vi "testVI.vi"() -> ()   [LabVIEW 2012]
uses:
  <vilib>/measure/NI_MABase.lvlib
  pgfPlotAxis_tdef.ctl
  pgfPlotPlot_tdef.ctl
  <vilib>/Waveform/WDTOps.llb/WDT Get Waveform Time Array DBL.vi
panel:
  in  "png?":bool=TRUE
  out "standard output":string
  out "output png":picture
  in  "amplitude":dbl=21.0 format="%0.2p"
  in  "frequency":dbl=3.0 format="%0.2p"
  in  "signal type":T1(ring)=enum."Triangle Wave"
  in  "add noise":bool=TRUE
  in  "number of points":dbl(slide)=44.4776119402985 scale=10.0..1000.0
  out "LaTeX output":string
  out "Waveform Graph":waveform(dbl)[](graph)=[{"t0"=timestamp(0 s since 1904-01-01), "dt"=0.02248322147651007, "Y"=[-1.546477433388504, 4.661984807620563, 7.8278201832138725, 11.001512342104604, 15.015062026967165, 15.512826662722626, 15.574358460996109, 13.290410667596724, 11.99348612908547, 8.588629763986237, 5.067512693167407, 1.258457503857374, -2.8810456117563374, -6.925805192568073, -10.545354256767709, -14.932883970541788, -13.577918727803066, -14.589587562163713, -11.46193309140618, -12.290200153543955, -9.437814005181771, -4.8264367558785795, -1.2386574847111085, 3.051340081786596, 6.950914289149695, 9.981049349063406, 12.35566247672647, 15.294188005780697, 14.350046666102049, 14.978056870639572, 13.443684958705374, 9.524808574601101, 5.281310569613, 0.09035510962493731, -3.3367521947681373, -5.625031359450402, -10.134935689127893, -12.522309407667565, -13.59685597158344, -14.168685301718552, -14.20184362459651, -12.77561767255461, -10.526530375259396, -7.10442228803309]}, {"t0"=timestamp(0 s since 1904-01-01), "dt"=0.001, "Y"=array[1000 elements]}]
  in  "Amplitude":dbl(slide)=15.016835016835017 scale=0.0..20.0
  # "first signal"
  # "second signal"
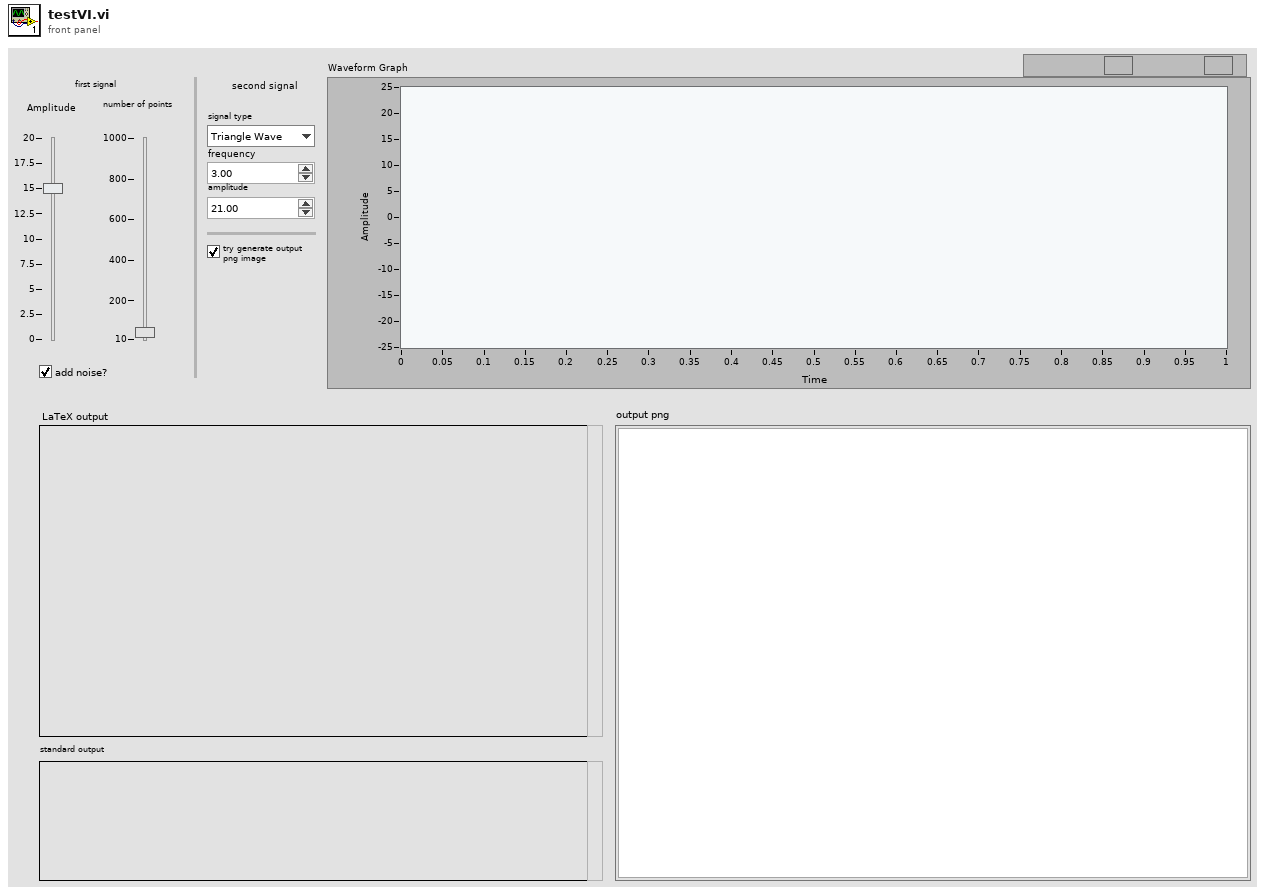
[diagram p1: front panel]
types:
  T1 = enum16{"Sine Wave", "Triangle Wave", "Square Wave", "Sawtooth Wave"}
  T2 = typedef "pgfPlotAxis_tdef.ctl" = cluster{"xmin":dbl, "xmax":dbl, "ymin":dbl, "ymax":dbl, "xLabel":string, "yLabel":string}
  T3 = typedef "pgfPlotPlot_tdef.ctl" = cluster{"LineStyle":u8, "LineWidth":u8, "PlotColor":u32, "Marker":u8, "PlotName":string, "x values":dbl[], "y values":dbl[]}
  T4 = typedef "LVBoundsTypeDef.ctl" = cluster{"Width":u32, "Height":u32}
  T5 = typedef "imagedata.ctl" = cluster{"image type":i32, "image depth":i32, "image":u8[], "mask":u8[], "colors":u32[], "Rectangle":cluster{"left":i16, "top":i16, "right":i16, "bottom":i16}}
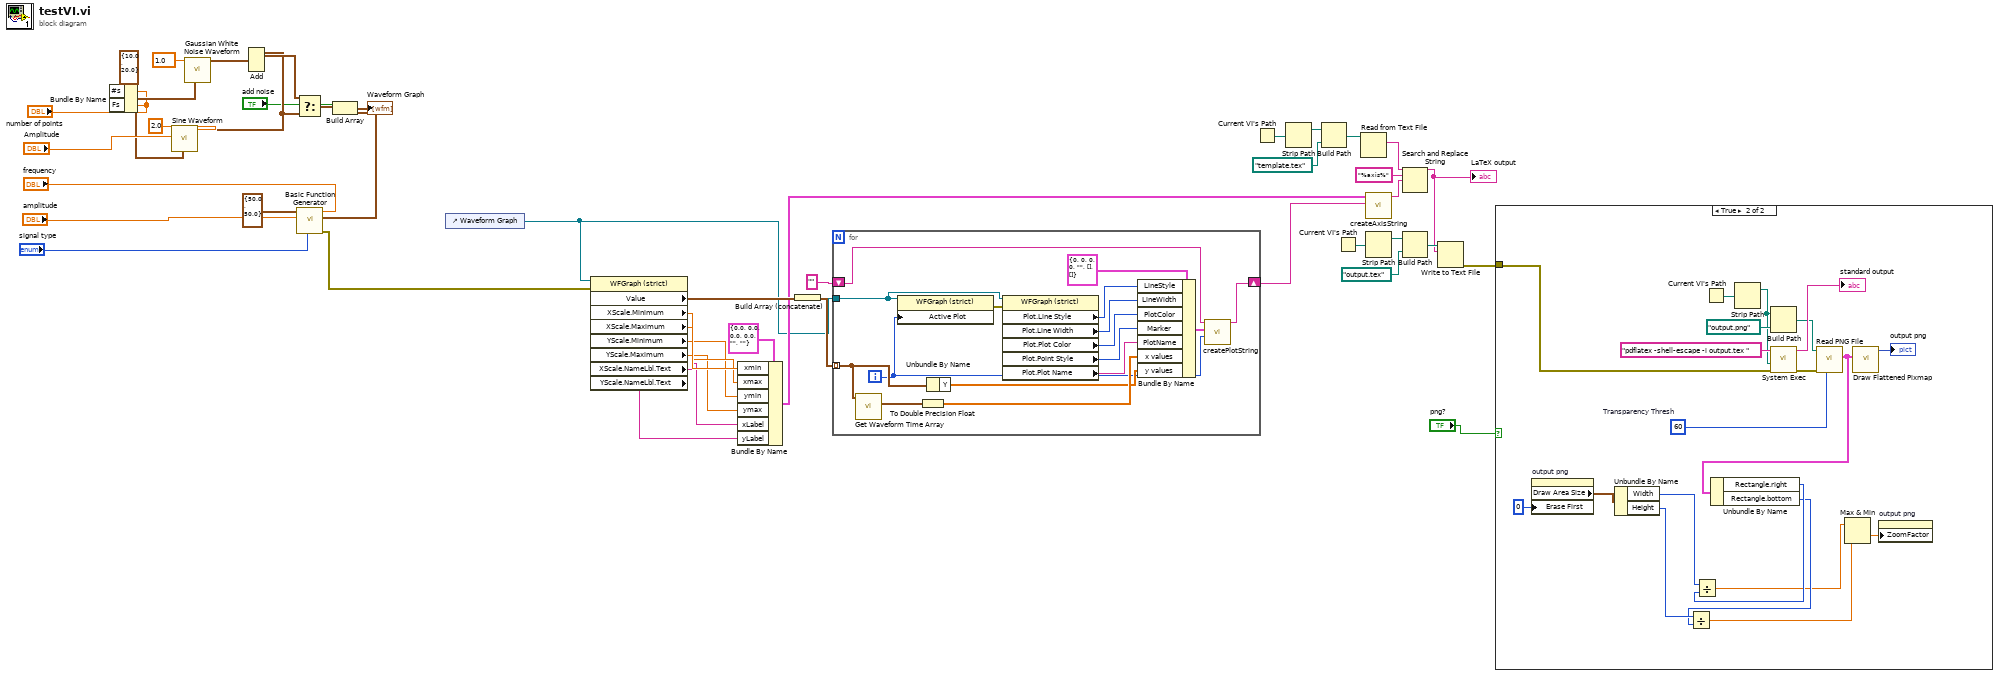
[diagram p0: block diagram]
diagram:
  n1 = Bundle By Name(cluster=cluster{"Fs":dbl, "#s":dbl} {"Fs"=10.0, "#s"=20.0} ("sampling info"), "#s"="number of points", "Fs"="number of points") -> (w14:cluster{"Fs":dbl, "#s":dbl})
  n2 = call <vilib>:"Sine Waveform.vi"("sampling info"=w14, "amplitude"="Amplitude", "frequency"=2.0 ("Frequency")) -> ("signal out"=w11:waveform(dbl))  [unwired: 7 in, 1 out]
  n3 = call <vilib>:"Gaussian White Noise Waveform.vi"("sampling info"=w14, "standard deviation"=1.0) -> ("signal out"=w45:waveform(dbl))  [unwired: 8 in, 1 out]
  n4 = Add(1:w45, 2:w11) -> (0:w12:waveform(dbl))  [unwired: 1 in, 1 out]
  n5 = Select(t=w12, s="add noise", f=w11) -> (s? t:f=w10:waveform(dbl))
  n6 = call <vilib>:"Basic Function Generator.vi"("sampling info"=cluster{"Fs":dbl, "#s":dbl} {"Fs"=50.0, "#s"=50.0}, "signal type"="signal type", "amplitude"="amplitude", "frequency"="frequency") -> ("error out"=w1:errorcluster, "signal out"=w8:waveform(dbl))  [unwired: 5 in, 1 out]
  n7 = Build Array(w10, w8) -> (→"Waveform Graph":waveform(dbl)[])
  n8 = control-ref of="Waveform Graph"() -> (w18:refnum<vi>)
  n9 = property class="WFGraph (strict)"(reference=w18, error in=w1) -> ("Value"=w33:waveform(dbl)[], "XScale.Minimum"=w28:dbl, "XScale.Maximum"=w27:dbl, "YScale.Minimum"=w26:dbl, "YScale.Maximum"=w25:dbl, "XScale.NameLbl.Text"=w24:string, "YScale.NameLbl.Text"=w23:string)  [unwired: 2 out]
  n10 = Bundle By Name(cluster=T2 {"xmin"=0.0, "xmax"=0.0, "ymin"=0.0, "ymax"=0.0, "xLabel"="", "yLabel"=""} ("Input"), "xmin"=w28, "xmax"=w27, "ymin"=w26, "ymax"=w25, "xLabel"=w24, "yLabel"=w23) -> (w22:T2)
  n11 = Build Array (concatenate)(w33) -> (w30:waveform(dbl)[])
  n12 = for {
    tunnel: w18 -> [w61]
    tunnel: w30 -> [w58] mode=indexing
    shift-right: [w57] -> w19
    shift-left: "" -> [w47]
    i -> [w46]
    n13 = call-poly <vilib>:"Get Waveform Time Array.vi"("waveform in"=w58) -> ("X array"=w60:timestamp[])  [unwired: 9 in, 1 out]
    n14 = property class="WFGraph (strict)"(reference=w61, "Active Plot"=w46) -> (error out=w59:errorcluster)  [unwired: 1 in, 1 out]
    n15 = To Double Precision Float(number=w60) -> (double precision float=w49:dbl[])
    n16 = Unbundle By Name(w58) -> ("Y"=w48:dbl[])
    n17 = property class="WFGraph (strict)"(reference=w61, error in=w59) -> ("Plot.Line Style"=w55:u8, "Plot.Line Width"=w54:u8, "Plot.Plot Color"=w50:u32, "Plot.Point Style"=w53:u8, "Plot.Plot Name"=w52:string)  [unwired: 2 out]
    n18 = Bundle By Name(cluster=T3 {"LineStyle"=0, "LineWidth"=0, "PlotColor"=0, "Marker"=0, "PlotName"="", "x values"=[], "y values"=[]}, "LineStyle"=w55, "LineWidth"=w54, "PlotColor"=w50, "Marker"=w53, "PlotName"=w52, "x values"=w49, "y values"=w48) -> (w51:T3)
    n19 = call "createPlotString.vi"("current plot number"=w46, "Plot Data"=w51, "plot string in"=w47) -> ("plot string out"=w57:string)  [unwired: 8 in]
  }
  n20 = Current VI's Path() -> (path=w41:path)
  n21 = Strip Path(path=w41) -> (stripped path=w40:path)  [unwired: 1 out]
  n22 = Build Path(base path=w40, name or relative path=path "template.tex" ("file (use dialog)")) -> (appended path=w38:path)
  n23 = Current VI's Path() -> (path=w35:path)
  n24 = Read from Text File(file (use dialog)=w38) -> (text=w31:string)  [unwired: 3 in, 3 out]
  n25 = call "createAxisString.vi"("PlotsString"=w19, "Input Data"=w22) -> ("AxisString"=w20:string)  [unwired: 9 in]
  n26 = Strip Path(path=w35) -> (stripped path=w36:path)  [unwired: 1 out]
  n27 = Search and Replace String(input string=w31, search string="%axis%", replace string=w20) -> (result string=w17:string)  [unwired: 5 in, 3 out]
  "LaTeX output" <- w17
  n28 = Build Path(base path=w36, name or relative path=path "output.tex" ("file (use dialog)")) -> (appended path=w34:path)
  n29 = Write to Text File(file (use dialog)=w34, text=w17) -> (error out=w3:errorcluster)  [unwired: 2 in, 2 out]
  n30 = case shown="True" "png?" {
    tunnel: w3 -> [_ w80]
    frame False {
    }
    frame True {
      w71 = u8 60  # Transparency Thresh
      n31 = property on="output png" class="Pict"("Erase First"=u8 0) -> ("Draw Area Size"=w70:T4)  [unwired: 2 in, 2 out]
      n32 = Unbundle By Name(w70) -> ("Width"=w69:u32, "Height"=w67:u32)
      n33 = Current VI's Path() -> (path=w76:path)
      n34 = Strip Path(path=w76) -> (stripped path=w72:path)  [unwired: 1 out]
      n35 = Build Path(base path=w72, name or relative path=path "output.png" ("file (use dialog)")) -> (appended path=w75:path)
      n36 = call <vilib>:"System Exec.vi"("error in (no error)"=w80, "working directory"=w72, "command line"="pdflatex -shell-escape -i output.tex ") -> ("error out"=w78:errorcluster, "standard output"=→"standard output":string)  [unwired: 5 in, 2 out]
      n37 = call <vilib>:"Read PNG File.vi"("Transparency Thresh"=w71, "error in (no error)"=w78, "path to PNG file"=w75) -> ("image data"=w73:T5)  [unwired: 6 in, 2 out]
      n38 = Unbundle By Name(w73) -> ("Rectangle.right"=w68:i16, "Rectangle.bottom"=w66:i16)
      n39 = Divide(x=w67, y=w66) -> (x/y=w64:dbl)
      n40 = Divide(x=w69, y=w68) -> (x/y=w65:dbl)
      n41 = Max & Min(x=w65, y=w64) -> (min(x,y)=w63:dbl)  [unwired: 1 out]
      n42 = call <vilib>:"Draw Flattened Pixmap.vi"("image data"=w73) -> ("new picture"=→"output png":picture)  [unwired: 8 in]
      n43 = property on="output png" class="Pict"("ZoomFactor"=w63) -> ()  [unwired: 2 in, 2 out]
    }
  }
